vi "Main.vi"() -> ()   [LabVIEW 2019]
uses:
  <vilib>/robotics/Controls/Attitude Indicator/Attitude Indicator.xctl
  <vilib>/Instr/_visa.llb/VISA Flush IO Buffer Mask.ctl
  <vilib>/MakerHub/LINX/Public/Peripherals/PWM/PWM Set Duty Cycle 1 Chan.vi
  <vilib>/MakerHub/LINX/Public/Peripherals/Digital/Digital Write 1 Chan.vi
  <vilib>/MakerHub/LINX/Public/Peripherals/Digital/Digital Write N Chans.vi
  <vilib>/MakerHub/LINX/Private/Local IO/LinxDigitalWrite.vi
  <vilib>/MakerHub/LINX/Public/Utilities/Check Channel.vi
  <vilib>/Instr/_visa.llb/VISA Configure Serial Port (Instr).vi
  <vilib>/MakerHub/LINX/Public/Utilities/Open Serial.vi
  <vilib>/MakerHub/LINX/Public/Peripherals/PWM/PWM Set Duty Cycle N Chans.vi
  <vilib>/MakerHub/LINX/Private/Utilties/Generate Error.vi
  <vilib>/MakerHub/LINX/LMH-LINX.lvlib
panel:
  in  "Both Stop":bool
  out "Meter":dbl(knob) scale=0.0..100.0
  in  "Serial Port":refnum<visa-resource-name>="N/A"
  in  "Motor Stop":bool
  in  "Speed":dbl(slide) scale=0.0..1.0
  in  "Forward":bool
  in  "backward":bool
  out "Angle of Attack":dbl
  out "Attitude Indicator":cluster{"Roll":dbl, "Pitch":dbl}(xcontrol)
  in  "COM Port":refnum<visa-resource-name>="COM5"
  out "Read Buffer":string
  out "Read Buffer (Debug)":string
  out "Elapsed Tme":timestamp format="%<%.3X>T"
  out "return count":u32
  in  "Attitude Stop":bool
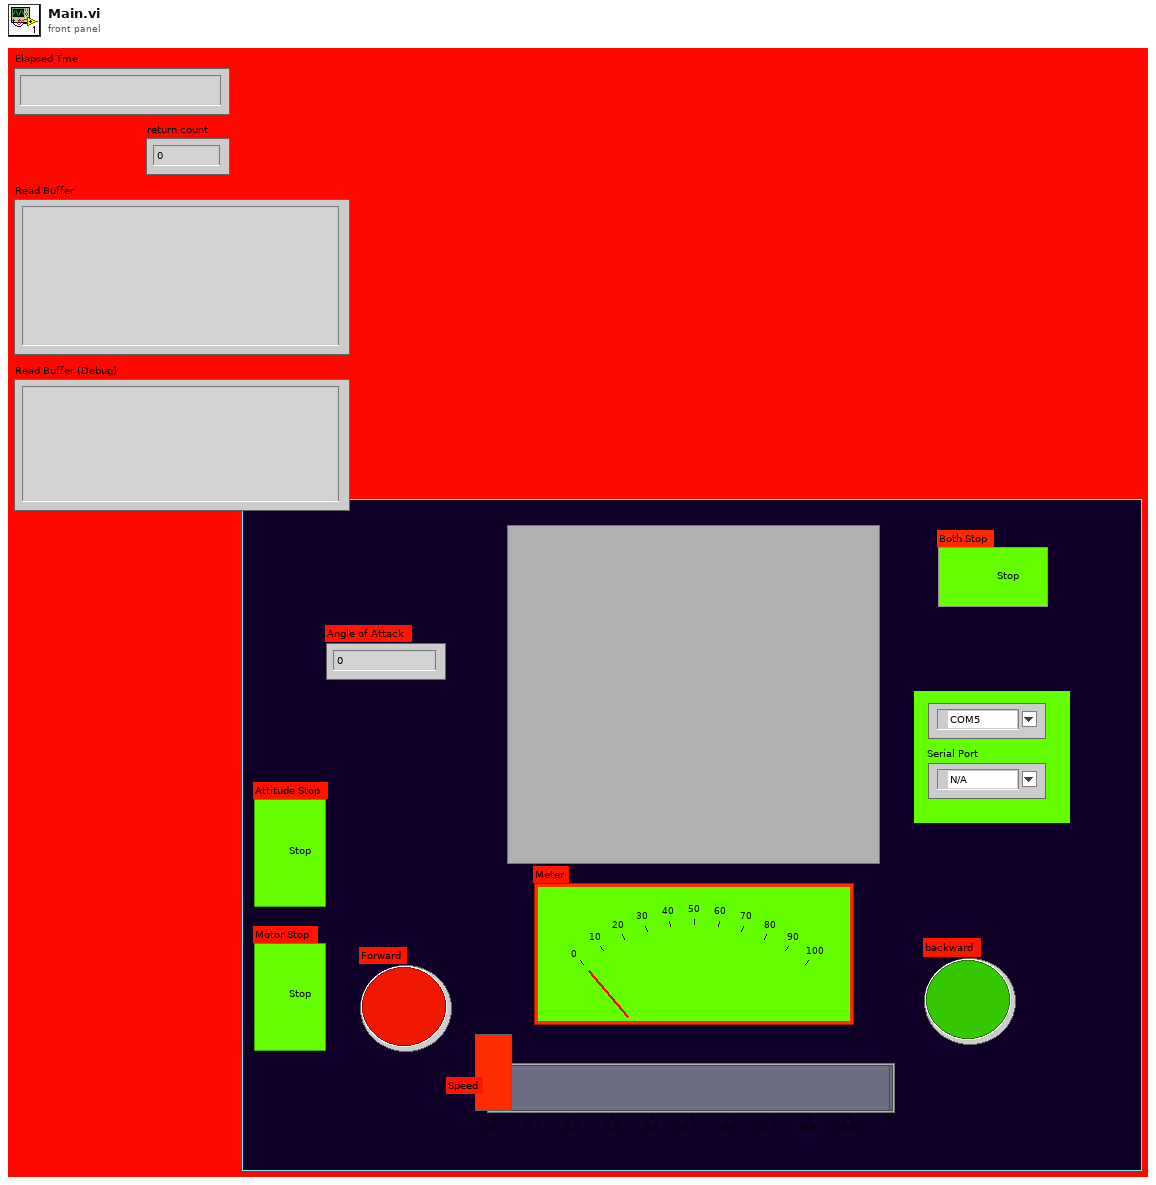
[diagram p1: front panel]
types:
  T1 = enum16{"Raw Acceleration", "Raw Gyro", "Complementy Filter", "Kalman Filter"}
  T2 = typedef "LMH-LINX.lvlib/LINX Ref.ctl" = cluster{"IO":T3, "Interface":T4, "LINX Device Config":T5}
  T3 = typedef "LMH-LINX.lvlib/Platform.ctl" = enum16{"Remote", "Local"}
  T4 = typedef "LMH-LINX.lvlib/Interface.ctl" = enum16{"Serial", "TCP"}
  T5 = typedef "LMH-LINX.lvlib/Device.lvlib/LINX Device Config.ctl" = cluster{"Interface":T4, "COM Port":refnum<visa-resource-name>, "TCP Configuration":T6, "Device Family":u8, "Device ID":u8, "Device Name":string, "TCP Ref":refnum<k5>, "Channels":T7}
  T6 = typedef "LMH-LINX.lvlib/Device.lvlib/TCP Config.ctl" = cluster{"IP Address":string, "Port":u16}
  T7 = typedef "LMH-LINX.lvlib/Channels.ctl" = cluster{"DI":u8[], "DO":u8[], "AI":u8[], "AO":u8[], "PWM":u8[], "QE":u8[], "UART":u8[], "I2C 2":u8[], "SPI":u8[], "CAN":u8[], "Servo":u8[], "AI Ref (V)":dbl, "AI Resolution (Bits)":u8, "AO Ref (V)":dbl, "AO Resolution (Bits)":u8}
  T8 = typedef "VISA Flush IO Buffer Mask.ctl" = u16
  T9 = cluster{"Numeric Control":dbl, "Numeric Control":dbl, "Numeric Control":dbl}
  T10 = cluster{"Numeric Control":dbl, "Numeric Control":dbl}
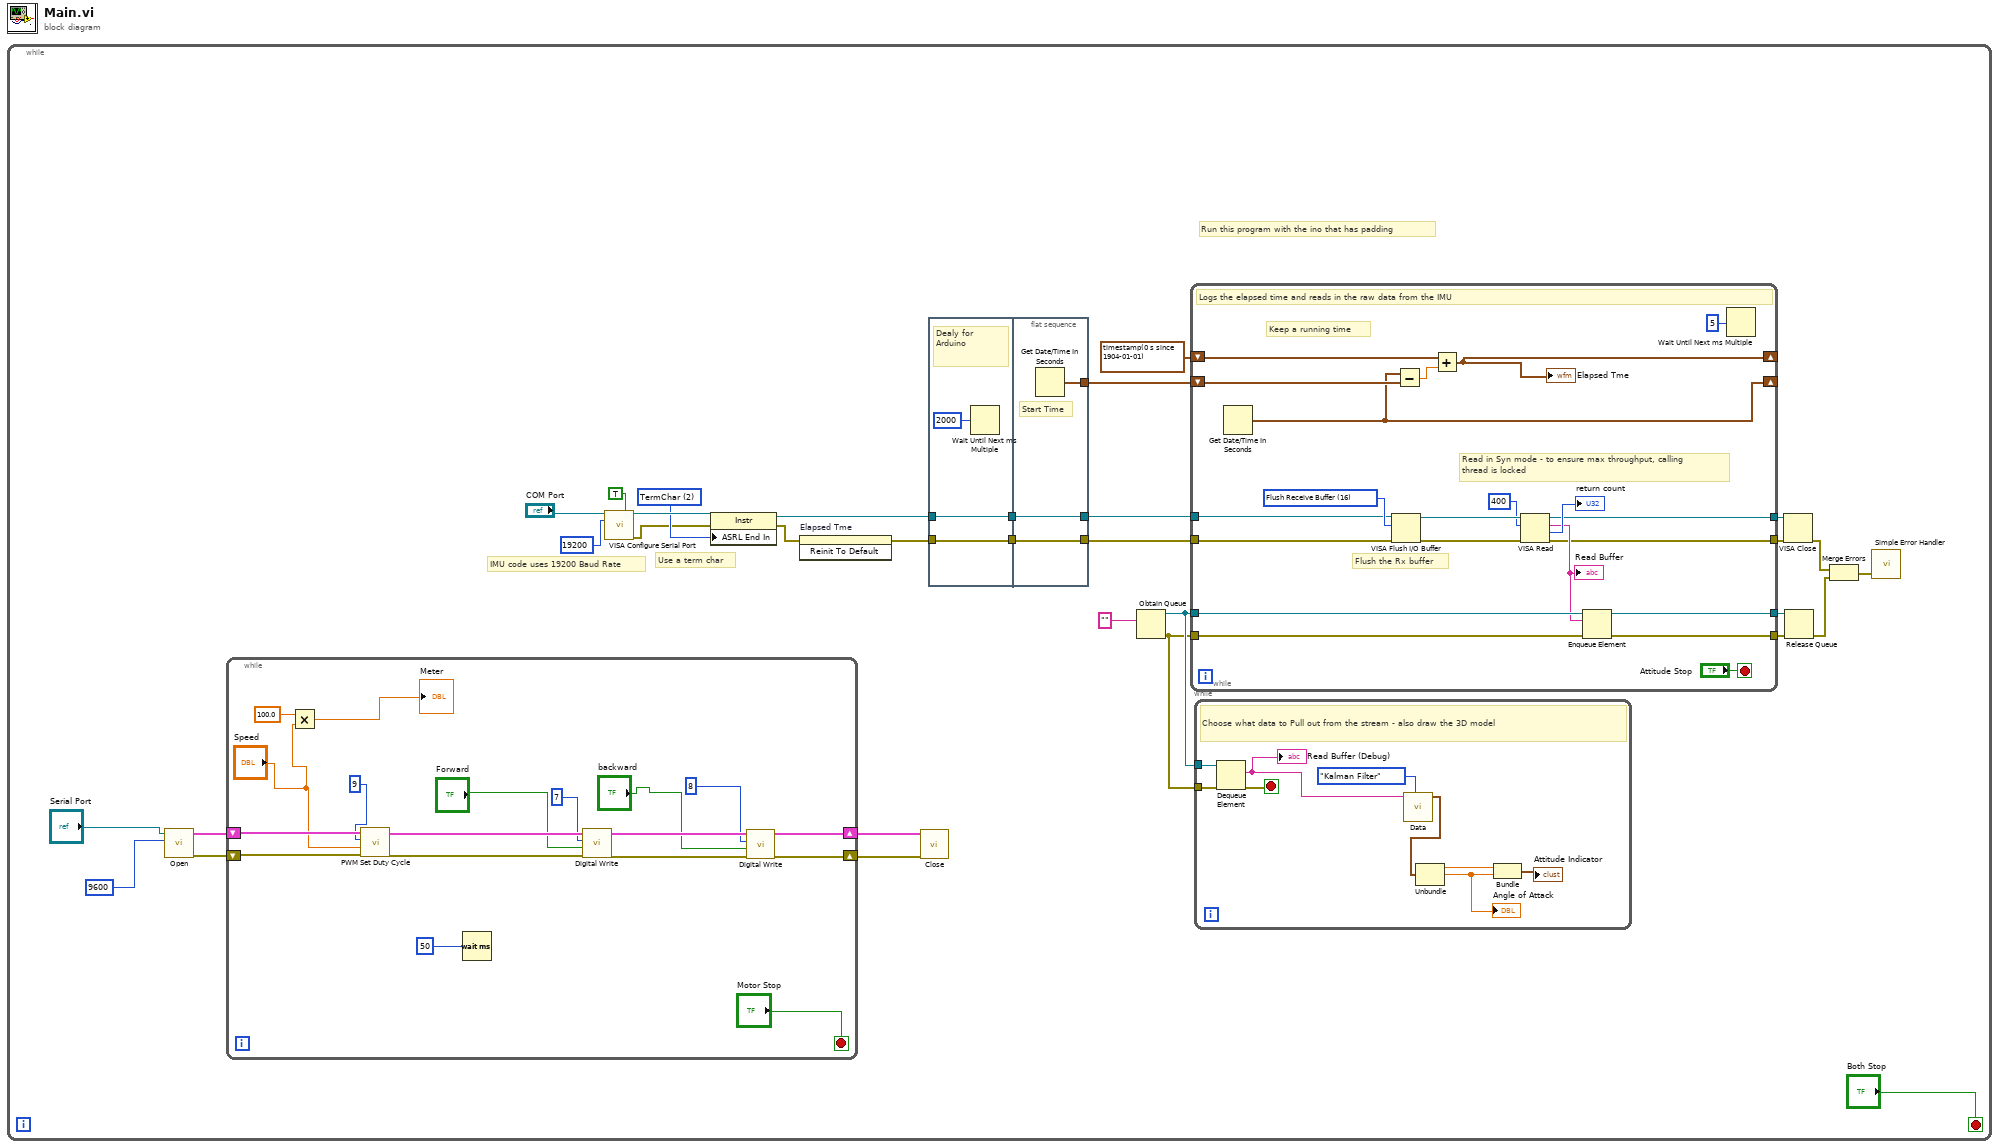
[diagram p0: block diagram]
diagram:
  n1 = while {
    stop <- "Both Stop" stop-if-true
    w23 = u16 2 items=["None", "Last Bit", "TermChar"] ("Serial Settings:End Mode for Reads")
    # "IMU code uses 19200 Baud Rate"
    # "Use a term char"
    # "Run this program with the ino that has padding"
    n2 = call-poly <vilib>:"Open.vi"("Baud Rate Override"=u32 9600, "Serial Port"="Serial Port") -> ("Error Out"=w7:errorcluster, "LINX Resource"=w8:T2)  [unwired: 7 in, 1 out]
    n3 = while {
      shift-right: [w44] -> w6
      shift-left: w8 -> [w49]
      shift-right: [w43] -> w5
      shift-left: w7 -> [w48]
      stop <- "Motor Stop" stop-if-true
      n4 = Multiply(x=100.0, y="Speed") -> (x*y=→"Meter":dbl)
      n5 = call-poly <vilib>:"PWM Set Duty Cycle.vi"("Error In"=w48, "Duty Cycle (0-1)"="Speed", "PWM Channel"=u8 9, "LINX Resource"=w49) -> ("Error Out"=w41:errorcluster, "LINX Resource"=w46:T2)  [unwired: 6 in]
      n6 = Wait (ms)(milliseconds to wait=u32 50 ("millisecond timer value")) -> ()  [unwired: 1 out]
      n7 = call-poly <vilib>:"Digital Write.vi"("Error In"=w41, "Output Value"="Forward", "DO Channel"=u8 7, "LINX Resource"=w46) -> ("Error Out"=w42:errorcluster, "LINX Resource"=w45:T2)  [unwired: 6 in]
      n8 = call-poly <vilib>:"Digital Write.vi"("Error In"=w42, "Output Value"="backward", "DO Channel"=u8 8, "LINX Resource"=w45) -> ("Error Out"=w43:errorcluster, "LINX Resource"=w44:T2)  [unwired: 6 in]
    }
    n9 = call-poly "VISA Configure Serial Port"("VISA resource name"="COM Port", "Enable Termination\nChar (T)"=TRUE ("Enable Termination\nChar (T)"), "baud rate (9600)"=u32 19200) -> ("VISA resource name out"=w24:refnum<visa-resource-name>, "error out"=w22:errorcluster)  [unwired: 11 in]
    n10 = property class="Instr"(reference=w24, error in=w22, "ASRL End In"=w23) -> (reference out=w9:refnum<visa-resource-name>, error out=w11:errorcluster)
    n11 = invoke on="Elapsed Tme" class="AbsTime (strict)" method="Reinit To Default"(error in=w11) -> (error out=w10:errorcluster)  [unwired: 2 in, 2 out]
    n12 = call <vilib>:"Close.vi"("Error In"=w5, "LINX Resource"=w6) -> ()  [unwired: 9 in, 1 out]
    n13 = flat-sequence {
      tunnel: w10 -> [w52]
      tunnel: w9 -> [w53]
      tunnel: [w53] -> w32
      tunnel: [w52] -> w31
      tunnel: [w56] -> w14
      tunnel: [w55] -> w13
      tunnel: [w54] -> w12
      tunnel: w32 -> [w56]
      tunnel: w31 -> [w55]
      frame #0 {
        # "Dealy for Arduino"
        n14 = Wait Until Next ms Multiple(millisecond multiple=u32 2000) -> ()  [unwired: 1 out]
      }
      frame #1 {
        # "Start Time"
        n15 = Get Date/Time In Seconds() -> (seconds since 1Jan1904=w54:timestamp)
      }
    }
    n16 = Obtain Queue(element data type="") -> (queue out=w26:refnum<queue>, error out=w18:errorcluster)  [unwired: 4 in, 1 out]
    n17 = while {
      tunnel: w14 -> [w71]
      tunnel: w13 -> [w72]
      shift-right: [w75] -> _
      shift-left: w12 -> [w80]
      shift-right: [w76] -> _
      shift-left: timestamp(0 s since 1904-01-01) -> [w79]
      tunnel: w26 -> [w74]
      tunnel: [w73] -> w27
      tunnel: [w69] -> w21
      tunnel: [w68] -> w20
      tunnel: [w67] -> w19
      tunnel: w18 -> [w66]
      stop <- "Attitude Stop" stop-if-true
      w81 = T8 16 items=["Flush Receive Buffer"=16, "Write Transmit Buffer to Device"=32, "Flush Receive Buffer (No I/O)"=64, "Flush Transmit Buffer"=128] ("Mask")
      # "Read in Syn mode - to ensure max throughput, calling\nthread is locked"
      # "Flush the Rx buffer"
      # "Keep a running time"
      # "Logs the elapsed time and reads in the raw data from the IMU"
      n18 = Get Date/Time In Seconds() -> (seconds since 1Jan1904=w75:timestamp)
      n19 = VISA Flush I/O Buffer(VISA resource name=w71, mask (16)=w81, error in (no error)=w72) -> (VISA resource name out=w84:refnum<visa-resource-name>, error out=w85:errorcluster)
      n20 = Subtract(x=w75, y=w80) -> (x-y=w77:dbl)
      n21 = Add(x=w79, y=w77) -> (x+y=w76:timestamp)
      "Elapsed Tme" <- w76
      n22 = VISA Read(VISA resource name=w84, byte count=u32 400, error in (no error)=w85) -> (VISA resource name out=w69:refnum<visa-resource-name>, read buffer=w70:string, return count=→"return count":u32, error out=w68:errorcluster)
      "Read Buffer" <- w70
      n23 = Enqueue Element(queue=w74, element=w70, error in (no error)=w66) -> (queue out=w73:refnum<queue>, error out=w67:errorcluster)  [unwired: 1 in, 1 out]
      n24 = Wait Until Next ms Multiple(millisecond multiple=u32 5) -> ()  [unwired: 1 out]
    }
    n25 = while {
      tunnel: w26 -> [w65]
      tunnel: w18 -> [w62]
      stop <- w64 stop-if-true
      # "Choose what data to Pull out from the stream - also draw the 3D model"
      n26 = Dequeue Element(queue=w65, error in (no error)=w62) -> (element=w63:string, error out=w64:errorcluster)  [unwired: 1 in, 2 out]
      "Read Buffer (Debug)" <- w63
      n27 = call "Data.vi"("Data Type"=T1."Kalman Filter", "Read Buffer"=w63) -> ("XYZ"=w60:T9)  [unwired: 8 in, 1 out]
      n28 = Unbundle(w60) -> ("Numeric Control"=w59:dbl, "Numeric Control"=w57:dbl)  [unwired: 1 out]
      "Angle of Attack" <- w57
      n29 = Bundle("Numeric Control"=w59, "Numeric Control"=w57) -> (→"Attitude Indicator":T10)  [unwired: 1 in]
    }
    n30 = VISA Close(VISA resource name=w21, error in (no error)=w20) -> (error out=w17:errorcluster)
    n31 = Release Queue(queue=w27, error in (no error)=w19) -> (error out=w16:errorcluster)  [unwired: 1 in, 2 out]
    n32 = Merge Errors(w17, w16) -> (w15:errorcluster)
    n33 = call <vilib>:"Simple Error Handler.vi"("error in (no error)"=w15) -> ()  [unwired: 4 in, 5 out]
  }
